vi "Measurement Template(Unary).vi"(8 "error in (no error)":errorcluster, 10 "stop":bool, 11 "measurement configuration":cluster{"Boolean":bool}) -> (0 "error out":errorcluster, 3 "measurement results":cluster{"Boolean":bool})   [LabVIEW 2021]
uses:
  Runtime/Clients/Measurement Service Client V2/RPC Messages/ni_measurementlink_measurement_v2_MeasureRequest.ctl
  Runtime/Clients/Measurement Service Client V2/RPC Messages/google_protobuf_Any.ctl
  Runtime/Clients/Measurement Service Client V2/RPC Messages/ni_measurementlink_PinMapContext.ctl
  35f71eb9-7158-4110-bfb1-6d749e6fa8f4.vi
  ef0035e8-05ef-469b-9be2-5e457b1f40d8.vi
  <vilib>/gRPC/LabVIEW gRPC Library/Server API/Translate Protobuf Error.vi
  <vilib>/AdvancedString/1D String Array to Delimited String.vi
  <vilib>/gRPC/LabVIEW gRPC Library/Server API/Server/Get Server DLL Path.vi
  <vilib>/gRPC/LabVIEW gRPC Library/grpc-lvsupport-release.lvlib
  Runtime/Clients/Measurement Service Client V2/Measurement Service Client V2.lvlib
  Runtime/Clients/Measurement Client V2/Client.lvlib
panel:
  in  "service class":string="Voltage Measurement_LabVIEW"
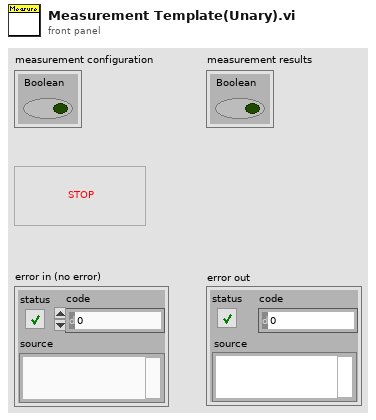
[diagram p1: front panel]
types:
  T1 = typedef "Measurement Service Client V2.lvlib/ni_measurementlink_measurement_v2_MeasureRequest.ctl" = cluster{"configuration_parameters":T2, "pin_map_context":T3}
  T2 = typedef "Measurement Service Client V2.lvlib/google_protobuf_Any.ctl" = cluster{"type_url":string, "value":u8[]}
  T3 = typedef "Measurement Service Client V2.lvlib/ni_measurementlink_PinMapContext.ctl" = cluster{"pin_map_id":string, "sites":i32[]}
  T4 = typedef "grpc-lvsupport-release.lvlib/grpcId.ctl" = u64
  T5 = typedef "grpc-lvsupport-release.lvlib/Message Metadata.ctl" = cluster{"Version":i32, "Name":string, "Type Url":string, "Elements":T6[], "Has Oneof":bool}
  T6 = typedef "grpc-lvsupport-release.lvlib/Message Element Metadata.ctl" = cluster{"Field Name":string, "Embedded Message Name":string, "Protobuf Index":i32, "MessageElementType":T7, "Repeated":bool, "Is in Oneof":bool, "Oneof Container Name":string}
  T7 = typedef "grpc-lvsupport-release.lvlib/Message Element Type.ctl" = enum32{"Int32Value", "FloatValue", "DoubleValue", "BoolValue", "StringValue", "MessageValue", "Int64Value", "UInt32Value", "UInt64Value", "EnumValue", "Bytes", "Fixed64", "Fixed32", "SFixed64", "SFixed32", "SInt64", "SInt32"}
  T8 = typedef "grpc-lvsupport-release.lvlib/Any.ctl" = cluster{"Type Url":string, "Bytes":u8[]}
  T9 = typedef "Measurement Service Client V2.lvlib/ni_measurementlink_measurement_v2_MeasureResponse.ctl" = cluster{"outputs":T2}
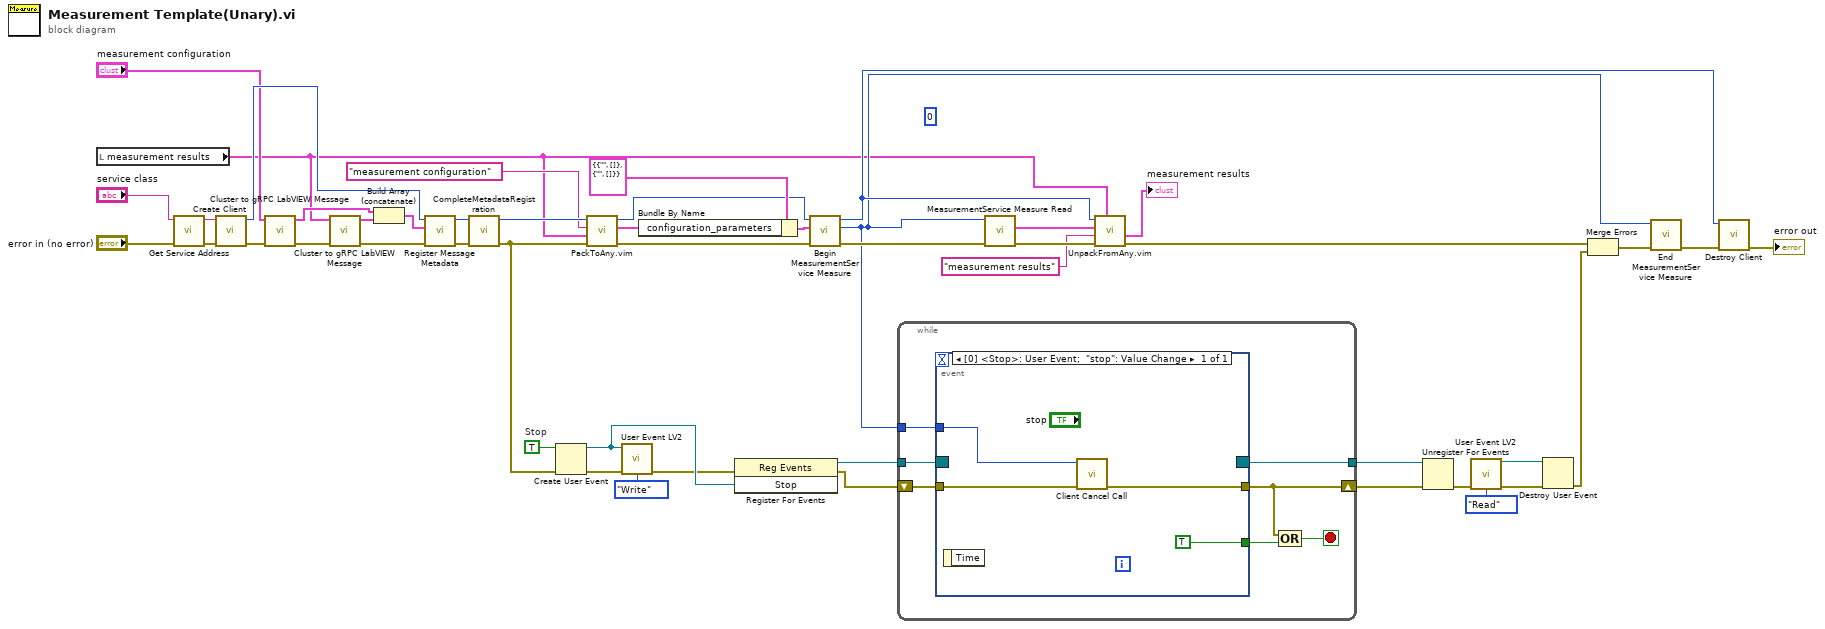
[diagram p0: block diagram]
diagram:
  (unwired) 0
  w24 = TRUE  # Stop
  n1 = local read "measurement results"() -> (w1:cluster{"Boolean":bool})
  n2 = call "Get Service Address.vi"("error in"="error in (no error)", "service to run"="service class") -> ("error out"=w38:errorcluster, "service address"=w36:string)  [unwired: 8 in]
  n3 = call "Create Client.vi"("error in"=w38, "address"=w36) -> ("error out"=w35:errorcluster, "gRPC ID Out"=w34:T4)  [unwired: 8 in]
  n4 = call <vilib>:"Cluster to gRPC LabVIEW Message.vi"("error in"=w35, "Cluster"="measurement configuration") -> ("error out"=w40:errorcluster, "gRPC Message Metadata []"=w48:T5[])  [unwired: 7 in, 1 out]
  n5 = call <vilib>:"Cluster to gRPC LabVIEW Message.vi"("error in"=w40, "Cluster"=w1) -> ("error out"=w39:errorcluster, "gRPC Message Metadata []"=w47:T5[])  [unwired: 7 in, 1 out]
  n6 = Build Array (concatenate)(w48, w47) -> (w46:T5[])
  n7 = call <vilib>:"Register Message Metadata.vi"("error in"=w39, "Messages"=w46, "gRPCid in"=w34) -> ("error out"=w45:errorcluster, "gRPCid out"=w33:T4)  [unwired: 7 in]
  n8 = call <vilib>:"CompleteMetadataRegistration.vi"("error in"=w45, "gRPC ID in"=w33) -> ("error out"=w23:errorcluster, "gRPC ID Out"=w32:T4)  [unwired: 8 in]
  n9 = Create User Event(user event datatype=w24, error in=w23) -> (user event=w20:refnum<user-event>, error out=w18:errorcluster)
  n10 = call "PackToAny.vim"("error in"=w23, "Data To Pack"=w1, "Message Type"="measurement configuration", "gRPCid in"=w32) -> ("error out"=w44:errorcluster, "Any"=w42:T8, "gRPCid out"=w28:u64)  [unwired: 5 in]
  n11 = call "User Event LV2.vi"("Stop event"=w20, "error in (no error)"=w18, "LV2 operations"=enum16{"Read", "Write"}."Write") -> ("error out"=w19:errorcluster)  [unwired: 11 in, 1 out]
  n12 = Bundle By Name(cluster=T1 {"configuration_parameters"={"type_url"="", "value"=[]}, "pin_map_context"={"pin_map_id"="", "sites"=[]}} ("Request Data"), "configuration_parameters"=w42) -> (w41:T1)
  n13 = register-events(error in=w19, w20) -> (reference out=w13:refnum<event-registration>, error out=w12:errorcluster)  [unwired: 1 in]
  n14 = call "Begin MeasurementService Measure.vi"("error in"=w44, "Request Data"=w41, "gRPC ID"=w28) -> ("error out"=w22:errorcluster, "Call Id Out"=w6:T4, "gRPC ID out"=w29:T4)  [unwired: 6 in]
  n15 = while {
    shift-right: [w54] -> w11
    shift-left: w12 -> [w55]
    tunnel: [w52] -> w10
    tunnel: w13 -> [w50]
    tunnel: w6 -> [w49]
    stop <- w51 stop-if-true
    n16 = event shown="[0] <Stop>: User Event;  \"stop\": Value Change" {
      selector: w50 -> [_]
      dyn-events: [_] -> w52
      timeout: _ -> [_]
      tunnel: w55 -> [w59]
      tunnel: [w58] -> w54
      tunnel: [TRUE] -> w53
      tunnel: w49 -> [w56]
      event User Event; "stop": Value Change {
        n17 = event-data() -> ()  [unwired: 1 in, 1 out]
        n18 = call <vilib>:"Client Cancel Call.vi"("error in"=w59, "Call ID in"=w56) -> ("error out"=w58:errorcluster)  [unwired: 7 in, 2 out]
      }
    }
    n19 = Compound Arithmetic op=OR(w54, w53) -> (w51:bool)
  }
  n20 = call "MeasurementService Measure Read.vi"("error in"=w22, "Call ID in"=w6) -> ("error out"=w4:errorcluster, "Response Data"=w5:T9)  [unwired: 6 in, 2 out]
  n21 = call "UnpackFromAny.vim"("Data Type"=w1, "error in"=w4, "Message Type"="measurement results", "Any"=w5, "gRPCid in"=w29) -> ("error out"=w9:errorcluster, "Unpacked Value"=→"measurement results":cluster{"Boolean":bool})  [unwired: 4 in, 1 out]
  n22 = Unregister For Events(event registration refnum=w10, error in=w11) -> (error out=w14:errorcluster)
  n23 = call "User Event LV2.vi"("error in (no error)"=w14, "LV2 operations"=enum16{"Read", "Write"}."Read") -> ("Stop event out"=w16:refnum<user-event>, "error out"=w15:errorcluster)  [unwired: 12 in]
  n24 = Destroy User Event(user event=w16, error in=w15) -> (error out=w7:errorcluster)
  n25 = Merge Errors(w9, w7) -> (w8:errorcluster)
  n26 = call "End MeasurementService Measure.vi"("error in"=w8, "Call ID in"=w6) -> ("error out"=w30:errorcluster)  [unwired: 8 in, 1 out]
  n27 = call "Destroy Client.vi"("error in"=w30, "gRPC ID"=w29) -> ("error out"=→"error out":errorcluster)  [unwired: 9 in]
